vi "Update Loading String.vi"(8 "error in (no error)":errorcluster, 9 "Items Total":i32, 10 "Items Scanned":i32, 11 "String Ref":refnum<vi>) -> (0 "error out":errorcluster)   [LabVIEW 2020, in "VI Properties Editor.lvlib"]
doc: "Updates the user-facing string identified by <B>String Ref</B> with the current numbers of <B>Items Scanned</B> compared to the number of <B>Items Total</B>."
uses:
  VI Properties Editor.lvlib
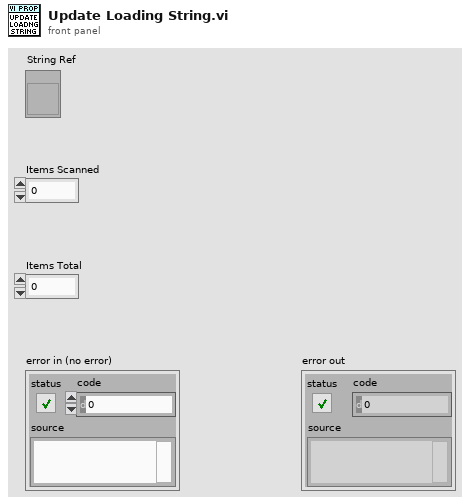
[diagram p1: front panel]
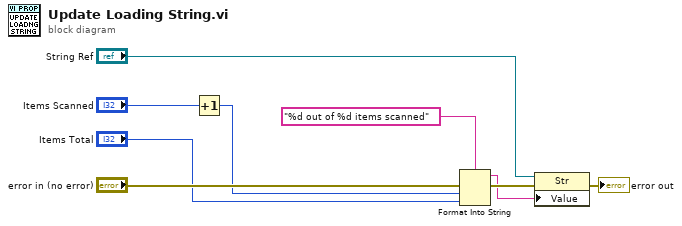
[diagram p0: block diagram]
diagram:
  n1 = Increment(x="Items Scanned") -> (x+1=w2:i32)
  n2 = Format Into String(format string="%d out of %d items scanned", error in="error in (no error)", w2, "Items Total") -> (resulting string=w1:string, error out=w9:errorcluster)  [unwired: 1 in]
  n3 = property class="Str"(reference="String Ref", error in=w9, "Value"=w1) -> (error out=→"error out":errorcluster)  [unwired: 1 out]
